vi "Stop and Empty FIFOs.vi"(8 "error in":errorcluster, 11 "Refnum in":T1) -> (0 "error out":errorcluster, 3 "FPGA VI Reference Out":T1)   [LabVIEW 2022 SP3]
doc: "Author: Scott Hannahs <sth@magnet.fsu.edu>\nCopyright 2018 Florida State University, All rights reserved."
uses:
  RT Controls/FPGA SCH Digitizer Ref.ctl
  <vilib>/Utility/error.llb/Error Cluster From Error Code.vi
  <vilib>/rvi/errors/niLvFpgaAdjustHostInterfaceError.vi
  <vilib>/rvi/interface/nirviReadWriteControl/nirviReadWriteControl.xnode
  <vilib>/rvi/interface/nirviMethod/nirviMethod.xnode
  <vilib>/rvi/errors/niLvFpgaMergeErrorWithErrorCode.vi
  <vilib>/FPGAPlugInAG/Dynamic/niLvFpga_ReadFifo_Dynamic.vi
  NiFpgaLv.dll
  <vilib>/rvi/interface/Simulation/niFpgaSimulationCallBeginRW.vi
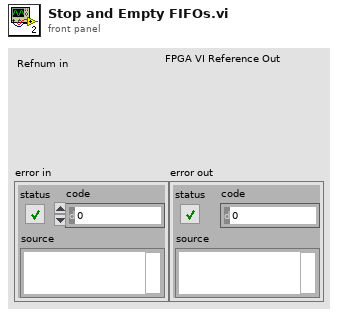
[diagram p1: front panel]
types:
  T1 = typedef "FPGA SCH Digitizer Ref.ctl" = refnum<k20>
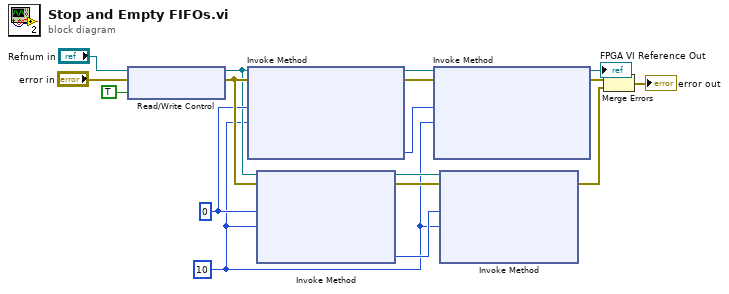
[diagram p0: block diagram]
diagram:
  w4 = 10 ("Timeout (ms)")
  w8 = u32 0 ("Number of Elements")
  n1 = xnode "Read/Write Control"("FPGA VI Reference In"="Refnum in", "error in"="error in", "Reset Digitizers"=TRUE ("Reset")) -> ("FPGA VI Reference Out"=w7:T1, "error out"=w12:errorcluster)
  n2 = xnode "Invoke Method"("FPGA VI Reference In"=w7, "error in"=w12, "Number of Elements"=w8, "Timeout (ms)"=w4) -> ("FPGA VI Reference Out"=w3:T1, "error out"=w11:errorcluster, "Elements Remaining"=w14:u32)  [unwired: 1 out]
  n3 = xnode "Invoke Method"("FPGA VI Reference In"=w7, "error in"=w12, "Number of Elements"=w8, "Timeout (ms)"=w4) -> ("FPGA VI Reference Out"=w9:T1, "error out"=w10:errorcluster, "Elements Remaining"=w13:u32)  [unwired: 1 out]
  n4 = xnode "Invoke Method"("FPGA VI Reference In"=w3, "error in"=w11, "Number of Elements"=w14, "Timeout (ms)"=w4) -> ("FPGA VI Reference Out"=→"FPGA VI Reference Out":T1, "error out"=w16:errorcluster)  [unwired: 2 out]
  n5 = xnode "Invoke Method"("FPGA VI Reference In"=w9, "error in"=w10, "Number of Elements"=w13, "Timeout (ms)"=w4) -> ("error out"=w15:errorcluster)  [unwired: 3 out]
  n6 = Merge Errors(w16, w15) -> (→"error out":errorcluster)
